vi "Digital Pass-Fail Boolean to Pass-Fail String.vi"(7 "Pass/Fail":bool) -> (8 "Pass/Fail String":string)   [LabVIEW 2019]
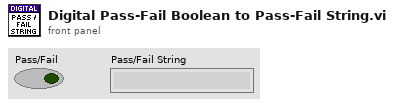
[diagram p1: front panel]
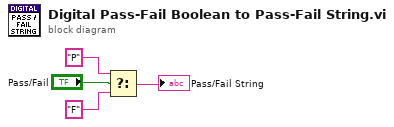
[diagram p0: block diagram]
diagram:
  n1 = Select(t="P", s="Pass/Fail", f="F") -> (s? t:f=→"Pass/Fail String":string)
